vi "Host - Find Slave Path.vi"(8 "error in (no error)":errorcluster, 11 "Item Ref in":T1 format="%.0x") -> (0 "error out":errorcluster, 1 "Target IP Address":string, 2 "Slave Ref":refnum<k21>, 3 "Item Ref out":T1=18446744073709551615 format="%.0x")   [LabVIEW 2019, in "SEECD System Explorer.lvlib"]
uses:
  SEECD System Explorer.lvlib
  <vilib>/NI VeriStand/Custom Device API/Custom Device Item Ref.ctl
  <vilib>/NI VeriStand/Custom Device API/Custom Device API.lvlib
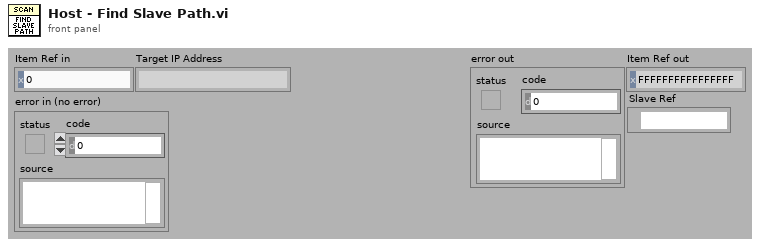
[diagram p1: front panel]
types:
  T1 = typedef "Custom Device API.lvlib/Custom Device Item Ref.ctl" = u64
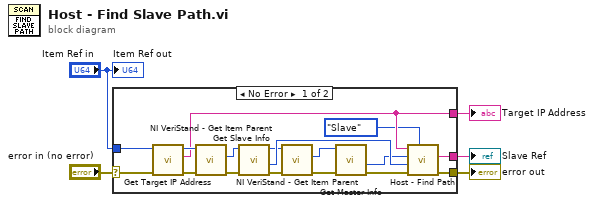
[diagram p0: block diagram]
diagram:
  n1 = case shown="No Error" "error in (no error)" {
    selector: "error in (no error)" -> [w11 w23]
    tunnel: "Item Ref in" -> [w12 _]
    tunnel: [w13 w23] -> w4
    tunnel: [w8 _] -> w2
    tunnel: [w6 _] -> w1
    frame No Error {
      n2 = call "Get Target IP Address.vi"("error in"=w11, "Item Ref in"=w12) -> ("error out"=w10:errorcluster, "Target IP Address"=w8:string, "Item Ref out"=w9:T1)  [unwired: 7 in]
      n3 = call <vilib>:"NI VeriStand - Get Item Parent.vi"("error in (no error)"=w10, "Item Ref in"=w9) -> ("error out"=w15:errorcluster, "Parent Ref"=w14:T1)  [unwired: 6 in, 2 out]
      n4 = call "Get Slave Info.vi"("error in (no error)"=w15, "Item Ref in"=w14) -> ("error out"=w17:errorcluster, "Slave #"=w22:u16, "Item Ref out"=w16:T1)  [unwired: 5 in, 2 out]
      n5 = call <vilib>:"NI VeriStand - Get Item Parent.vi"("error in (no error)"=w17, "Item Ref in"=w16) -> ("error out"=w19:errorcluster, "Parent Ref"=w18:T1)  [unwired: 6 in, 2 out]
      n6 = call "Get Master Info.vi"("error in (no error)"=w19, "Item Ref in"=w18) -> ("error out"=w20:errorcluster, "Master #"=w21:u32)  [unwired: 6 in, 2 out]
      n7 = call "Host - Find Path.vi"("Type"=enum16{"Slave", "Master"}."Slave", "error in (no error)"=w20, "Slave Index"=w22, "Master Index"=w21, "serverName"=w8) -> ("error out"=w13:errorcluster, "Path"=w6:string)  [unwired: 5 in]
    }
    frame Error {
    }
  }
  "error out" <- w4
  "Target IP Address" <- w2
  "Slave Ref" <- w1
  "Item Ref out" <- "Item Ref in"
